vi "Last Conf Save.vi"(0 "Conf Dir":path, 2 "Conf File":path) -> (9 "error out":errorcluster)   [LabVIEW 2019, in "Settings.lvlib"]
uses:
  Settings.lvlib
  <vilib>/Utility/config.llb/Write Key (String).vi
  <vilib>/Utility/config.llb/NI_LVConfig.lvlib
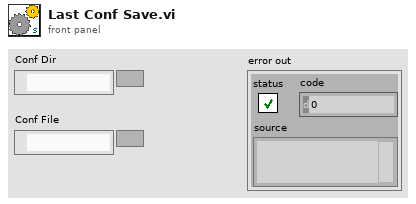
[diagram p1: front panel]
types:
  T1 = typedef "NI_LVConfig.lvlib/Config Data RefNum.ctl" = refnum<k1>
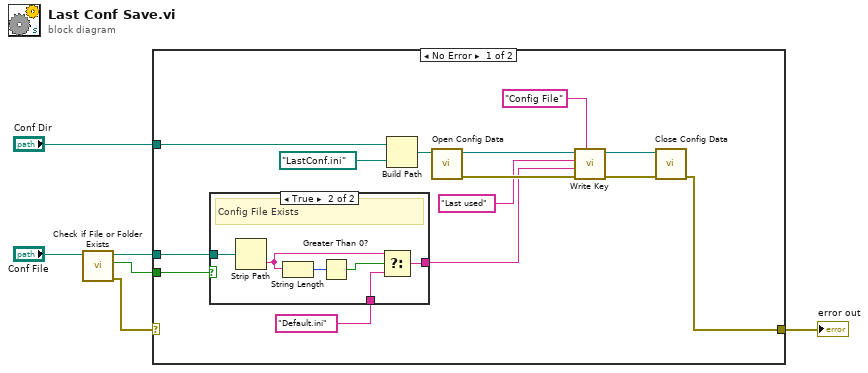
[diagram p0: block diagram]
diagram:
  n1 = call <vilib>:"Check if File or Folder Exists.vi"("path"="Conf File") -> ("error out"=w5:errorcluster, "file or folder exists?"=w4:bool, "dup path"=w3:path)  [unwired: 8 in]
  n2 = case shown="No Error" w5 {
    selector: w5 -> [_ w28]
    tunnel: w4 -> [w20 _]
    tunnel: w3 -> [w19 _]
    tunnel: [w10 w28] -> w2
    tunnel: "Conf Dir" -> [w7 _]
    frame No Error {
      n3 = case shown="True" w20 {
        tunnel: w19 -> [_ w27]
        tunnel: [w21 w26] -> w8
        tunnel: "Default.ini" -> [w21 w22]
        frame False {
          # "No Config File"
        }
        frame True {
          # "Config File Exists"
          n4 = Strip Path(path=w27) -> (name=w24:string)  [unwired: 1 out]
          n5 = String Length(string=w24) -> (length=w25:i32)
          n6 = Greater Than 0?(x=w25) -> (x > 0?=w23:bool)
          n7 = Select(t=w24, s=w23, f=w22) -> (s? t:f=w26:string)
        }
      }
      n8 = Build Path(base path=w7, name or relative path=path "LastConf.ini") -> (appended path=w18:path)
      n9 = call <vilib>:"Open Config Data.vi"("configuration file path"=w18) -> ("error out"=w17:errorcluster, "refnum"=w16:T1)  [unwired: 8 in, 1 out]
      n10 = call-poly <vilib>:"Write Key.vi"("section"="Config File", "error in (no error)"=w17, "value"=w8, "key"="Last used", "refnum"=w16) -> ("error out"=w11:errorcluster, "refnum out"=w12:T1)  [unwired: 4 in, 1 out]
      n11 = call <vilib>:"Close Config Data.vi"("error in (no error)"=w11, "refnum"=w12) -> ("error out"=w10:errorcluster)  [unwired: 8 in, 1 out]
    }
    frame Error {
    }
  }
  "error out" <- w2
